vi "Destructor.vi"(8 "error in":errorcluster, 11 "Defect":refnum<class "Defect.lvclass">) -> (0 "error out":errorcluster)   [LabVIEW 2021, in "ProligentXMLGenerator.lvlib" / "Defect.lvclass"]
uses:
  Defect.lvclass
  Defect.lvclass/Defect.ctl
  Model/UserComment/UserComment.lvclass
  Model/CustomData/CustomData.lvclass
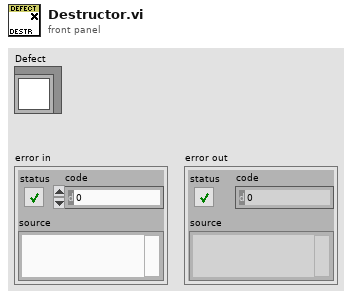
[diagram p1: front panel]
types:
  T1 = typedef "ProligentXMLGenerator.lvlib/Defect.lvclass/Data.ctl" = cluster{"Name":string, "Comments":refnum<class "UserComment.lvclass">[], "CustomData":refnum<class "CustomData.lvclass">, "DefectId":refnum<class "Guid.lvclass">, "OpenTime":refnum<class "DateTime.lvclass">, "TimeZoneInfoId":string}
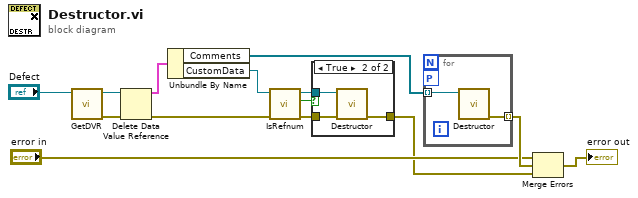
[diagram p0: block diagram]
diagram:
  n1 = call "GetDVR.vi"("Defect"="Defect") -> ("error out"=w10:errorcluster, "DVRReference"=w11:refnum<data-value>)  [unwired: 9 in]
  n2 = Delete Data Value Reference(data value reference=w11, error in=w10) -> (data value=w9:T1, error out=w1:errorcluster)
  n3 = Unbundle By Name(w9) -> ("Comments"=w7:refnum<class "UserComment.lvclass">[], "CustomData"=w4:refnum<class "CustomData.lvclass">)
  n4 = call "IsRefnum.vi"("error in"=w1, "CustomDataType in"=w4) -> ("error out"=w6:errorcluster, "IsRefnum"=w5:bool, "CustomDataType out"=w2:refnum<class "CustomData.lvclass">)  [unwired: 7 in]
  n5 = case shown="True" w5 {
    tunnel: w6 -> [w15 w18]
    tunnel: [w15 w17] -> w3
    tunnel: w2 -> [_ w16]
    frame False {
    }
    frame True {
      n6 = call "Destructor.vi"("error in"=w18, "CustomDataType"=w16) -> ("error out"=w17:errorcluster)  [unwired: 9 in]
    }
  }
  n7 = for {
    tunnel: w7 -> [w20] mode=indexing
    tunnel: [w19] -> w14 mode=indexing
    workers-P: _ -> [_]
    n8 = call "Destructor.vi"("UserComment"=w20) -> ("error out"=w19:errorcluster)  [unwired: 10 in]
  }
  n9 = Merge Errors("error in", w14, w3) -> (→"error out":errorcluster)
